vi "Initialize Hardware.vi"(6 "logging enabled":bool, 7 "minor frame period (us)":dbl, 8 "error in":errorcluster, 9 "starting buffer index":u16, 10 "1553 configuration":T4, 11 "aim hardware parameters":T12) -> (0 "error out":errorcluster, 1 "rt subaddress to buffer id map":T2, 2 "bc subaddress to buffer id map":T1, 3 "module reference":T11)   [LabVIEW 2020, in "AIM MIL-STD-1553 Engine.lvlib" / "Implementation.lvlib" / "Shared Resources.lvclass"]
uses:
  Shared Resources.lvclass
  Shared/AIM Hardware Parameters.ctl
  Shared/Initialization Method.ctl
  Shared/Bus Selection.ctl
  Shared/Coupling Mode.ctl
  Shared/Timing Mode.ctl
  Hardware API/Module Reference.ctl
  Custom Device/1553 Configuration.ctl
  Custom Device/Bus Controller Configuration.ctl
  Custom Device/Major Frame Configuration.ctl
  Custom Device/Minor Frame Configuration.ctl
  Custom Device/Acyclic Frame Configuration.ctl
  Custom Device/Message Configuration.ctl
  Custom Device/Remote Terminal Configuration.ctl
  Shared/Direction.ctl
  RT Subaddress to Buffer ID Map.ctl
  BC Subaddress to Buffer ID Map.ctl
  <instrlib>/_AIM MIL-STD-1553/AIM Controls/1553 BC Transfer Settings.ctl
  Hardware API/AIM MIL-STD-1553 Hardware API.lvlib
  <vilib>/NI VeriStand/Custom Device Tools/Custom Device Utility Library/Custom Device Utility Library.lvlib
  Custom Device/Custom Device.lvlib
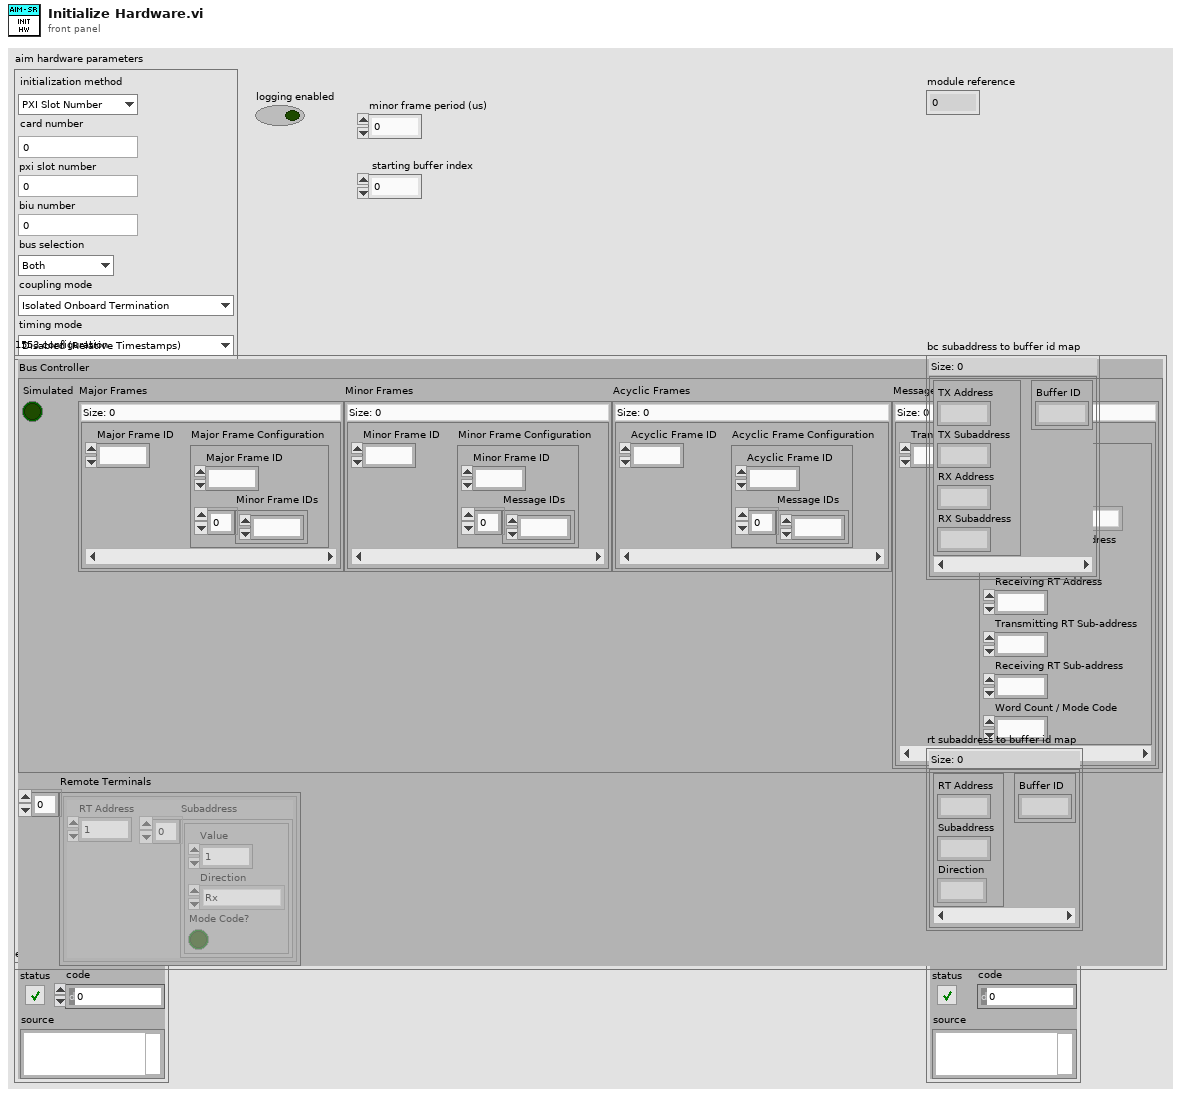
[diagram p1: front panel]
types:
  T1 = typedef "AIM MIL-STD-1553 Engine.lvlib/Implementation.lvlib/Shared Resources.lvclass/BC Subaddress to Buffer ID Map.ctl" = map{cluster{"TX Address":u8, "TX Subaddress":u8, "RX Address":u8, "RX Subaddress":u8}, cluster{"Buffer ID":u16}}
  T2 = typedef "AIM MIL-STD-1553 Engine.lvlib/Implementation.lvlib/Shared Resources.lvclass/RT Subaddress to Buffer ID Map.ctl" = map{cluster{"RT Address":u8, "Subaddress":u8, "Direction":T3}, cluster{"Buffer ID":u16}}
  T3 = typedef "Direction.ctl" = enum16{"Rx", "Tx"}
  T4 = typedef "AIM MIL-STD-1553 Engine.lvlib/Custom Device.lvlib/1553 Configuration.ctl" = cluster{"Bus Controller":T5, "Remote Terminals":T10[]}
  T5 = typedef "AIM MIL-STD-1553 Engine.lvlib/Custom Device.lvlib/Bus Controller Configuration.ctl" = cluster{"Simulated":bool, "Major Frames":map{u8, T6}, "Minor Frames":map{u8, T7}, "Acyclic Frames":map{u8, T8}, "Messages":map{u16, T9}}
  T6 = typedef "AIM MIL-STD-1553 Engine.lvlib/Custom Device.lvlib/Major Frame Configuration.ctl" = cluster{"Major Frame ID":u8, "Minor Frame IDs":u8[]}
  T7 = typedef "AIM MIL-STD-1553 Engine.lvlib/Custom Device.lvlib/Minor Frame Configuration.ctl" = cluster{"Minor Frame ID":u8, "Message IDs":u16[]}
  T8 = typedef "AIM MIL-STD-1553 Engine.lvlib/Custom Device.lvlib/Acyclic Frame Configuration.ctl" = cluster{"Acyclic Frame ID":u8, "Message IDs":u16[]}
  T9 = typedef "AIM MIL-STD-1553 Engine.lvlib/Custom Device.lvlib/Message Configuration.ctl" = cluster{"Transfer ID":u16, "Transfer Type":enum16{"BC to RT transfer", "RT to BC transfer", "RT to RT transfer"}, "Transmitting RT Address":u8, "Receiving RT Address":u8, "Transmitting RT Sub-address":u8, "Receiving RT Sub-address":u8, "Word Count / Mode Code":u8}
  T10 = typedef "AIM MIL-STD-1553 Engine.lvlib/Custom Device.lvlib/Remote Terminal Configuration.ctl" = cluster{"RT Address":u8, "Subaddress":cluster{"Value":u8, "Direction":T3, "Mode Code?":bool}[]}
  T11 = typedef "AIM MIL-STD-1553 Hardware API.lvlib/Module Reference.ctl" = u32
  T12 = typedef "AIM Hardware Parameters.ctl" = cluster{"initialization method":T13, "card number":i32, "pxi slot number":i32, "biu number":i32, "bus selection":T14, "coupling mode":T15, "timing mode":T16}
  T13 = typedef "Initialization Method.ctl" = enum16{"PXI Slot Number", "Card Number"}
  T14 = typedef "Bus Selection.ctl" = enum16{"Both", "Primary", "Secondary"}
  T15 = typedef "Coupling Mode.ctl" = enum16{"Isolated Onboard Termination", "Transformer Coupled", "Direct Coupled", "External with Onboard Termination", "Onboard Digital Wrap-around"}
  T16 = typedef "Timing Mode.ctl" = enum16{"Disabled (Relative Timestamps)", "IRIG (Internal System Time)", "IRIG (External Timing Source)"}
  T17 = typedef "1553 BC Transfer Settings.ctl" = cluster{"Start Mode (immediate)":enum16{"undefined", "Immediate", "External trigger", "Mode code dynamic bus control", "External pulse", "Setup for fast start", "Fast start", "Start instruction table", "Continue instruction table"}, "Count (0 = infinite)":u32, "Minor Frame Time (1 msec)":sgl, "Start Address (0)":u32}
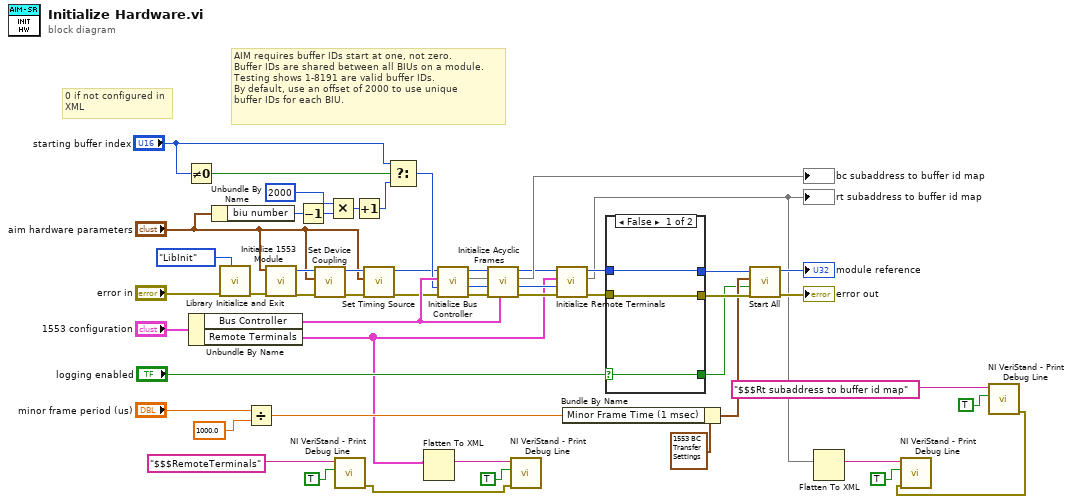
[diagram p0: block diagram]
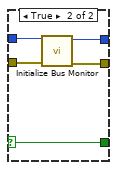
[diagram p2: hidden frame]
diagram:
  # "0 if not configured in XML"
  # "AIM requires buffer IDs start at one, not zero.\nBuffer IDs are shared between all BIUs on a module.\nTesting shows 1-8191 are valid buffer IDs.\nBy default, use an offset of 2000 to use unique\nbuffer IDs for each BIU."
  n1 = Not Equal To 0?(x="starting buffer index") -> (x != 0?=w22:bool)
  n2 = Unbundle By Name("1553 configuration") -> ("Bus Controller"=w33:T5, "Remote Terminals"=w12:T10[])
  n3 = Unbundle By Name("aim hardware parameters") -> ("biu number"=w45:i32)
  n4 = call "Library Initialize and Exit.vi"("action"=enum16{"LibInit", "LibExit"}."LibInit", "error in"="error in") -> ("error out"=w52:errorcluster)  [unwired: 8 in, 1 out]
  n5 = Divide(x="minor frame period (us)", y=1000.0) -> (x/y=w23:dbl)
  n6 = call "Initialize 1553 Module.vi"("error in"=w52, "hardware parameters"="aim hardware parameters") -> ("error out"=w49:errorcluster, "module handle out"=w50:u32)  [unwired: 8 in]
  n7 = Decrement(x=w45) -> (x-1=w43:i32)
  n8 = call "Set Device Coupling.vi"("error in"=w49, "aim hardware parameters"="aim hardware parameters", "module handle"=w50) -> ("error out"=w16:errorcluster, "module handle out"=w17:u32)  [unwired: 7 in]
  n9 = Multiply(x=2000, y=w43) -> (x*y=w42:i32)
  n10 = call <vilib>:"NI VeriStand - Print Debug Line.vi"("Add to log file? (F)"=TRUE, "Message"="$$$RemoteTerminals") -> ("error out"=w4:errorcluster)  [unwired: 9 in]
  n11 = Increment(x=w42) -> (x+1=w21:i32)
  n12 = call "Set Timing Source.vi"("error in"=w16, "hardware parameters"="aim hardware parameters", "module handle"=w17) -> ("error out"=w15:errorcluster, "module handle out"=w14:u32)  [unwired: 7 in]
  n13 = Select(t="starting buffer index", s=w22, f=w21) -> (s? t:f=w19:i32)
  n14 = Flatten To XML(6:w12) -> (2:w11:string)
  n15 = call "Initialize Bus Controller.vi"("error in"=w15, "next available buffer id"=w19, "bus controller"=w33, "module handle"=w14) -> ("error out"=w37:errorcluster, "next available buffer id out"=w38:u16, "bc address to buffer id map"=w40:T1, "module handle out"=w39:u32)  [unwired: 4 in]
  n16 = call "Initialize Acyclic Frames.vi"("bus controller"=w33, "error in"=w37, "next available buffer id"=w38, "bc address to \nbuffer id map"=w40, "module handle"=w39) -> ("error out"=w34:errorcluster, "next available buffer id out"=w35:u16, "bc address to buffer id map out"=→"bc subaddress to buffer id map":T1, "module handle out"=w36:u32)  [unwired: 3 in]
  n17 = call <vilib>:"NI VeriStand - Print Debug Line.vi"("error in (no error)"=w4, "Add to log file? (F)"=TRUE, "Message"=w11) -> ()  [unwired: 8 in, 1 out]
  n18 = call "Initialize Remote Terminals.vi"("error in"=w34, "next available buffer id"=w35, "remote terminals"=w12, "module handle"=w36) -> ("error out"=w31:errorcluster, "rt address to buffer id map"=w7:T2, "module handle out"=w32:u32)  [unwired: 4 in, 1 out]
  "rt subaddress to buffer id map" <- w7
  n19 = Bundle By Name(cluster=T17 {"Start Mode (immediate)"=enum."Immediate", "Count (0 = infinite)"=0, "Minor Frame Time (1 msec)"=0.001, "Start Address (0)"=0} ("bus controller transfer settings (default)"), "Minor Frame Time (1 msec)"=w23) -> (w26:T17)
  n20 = case shown="False" "logging enabled" {
    selector: "logging enabled" -> [w54 w57]
    tunnel: w32 -> [w55 w61]
    tunnel: w31 -> [w56 w60]
    tunnel: [w56 w59] -> w30
    tunnel: [w55 w58] -> w29
    tunnel: [w54 w57] -> w18
    frame False {
    }
    frame True {
      n21 = call "Initialize Bus Monitor.vi"("error in"=w60, "module handle"=w61) -> ("error out"=w59:errorcluster, "module handle out"=w58:u32)  [unwired: 8 in]
    }
  }
  n22 = call "Start All.vi"("error in"=w30, "logging configured?"=w18, "bus controller transfer settings (default)"=w26, "module handle"=w29) -> ("error out"=→"error out":errorcluster, "module handle out"=→"module reference":u32)  [unwired: 6 in]
  n23 = Flatten To XML(6:w7) -> (2:w8:string)
  n24 = call <vilib>:"NI VeriStand - Print Debug Line.vi"("Add to log file? (F)"=TRUE, "Message"="$$$Rt subaddress to buffer id map") -> ("error out"=w1:errorcluster)  [unwired: 9 in]
  n25 = call <vilib>:"NI VeriStand - Print Debug Line.vi"("error in (no error)"=w1, "Add to log file? (F)"=TRUE, "Message"=w8) -> ()  [unwired: 8 in, 1 out]
